vi "Dice Application.vi"() -> ()   [LabVIEW 2024]
uses:
  <vilib>/numeric/Random Number (Range) U64.vi
  <vilib>/numeric/sub_Random U32.vi
panel:
  out "Waveform Chart":u32(graph)
  in  "Throw Dice":bool
  in  "Stop":bool
  out "Dice":u32
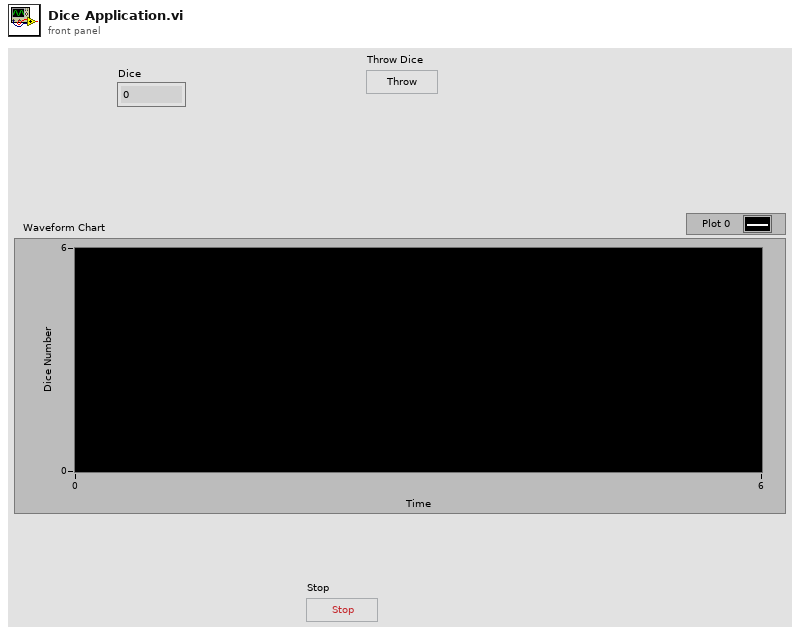
[diagram p1: front panel]
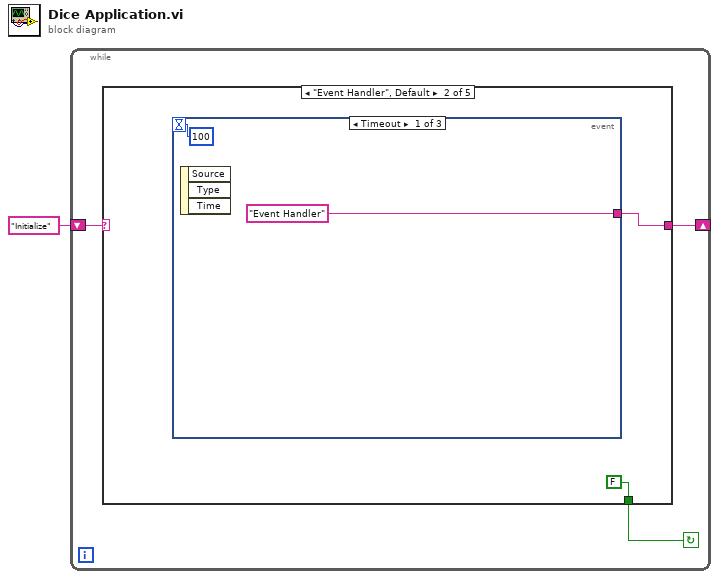
[diagram p0: block diagram]
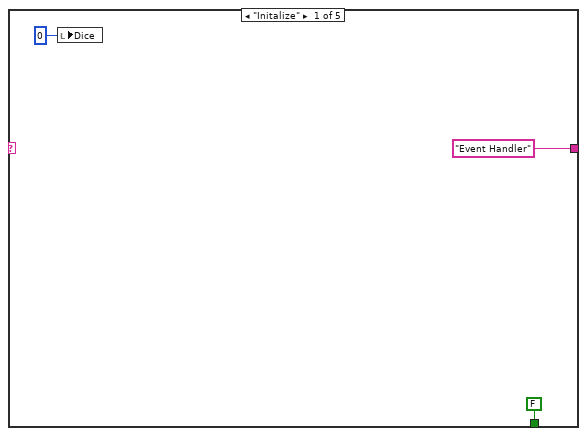
[diagram p2: hidden frame]
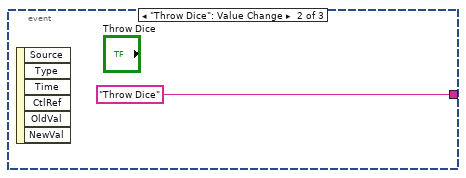
[diagram p3: hidden frame]
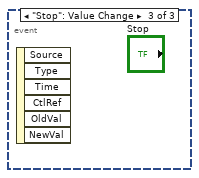
[diagram p4: hidden frame]
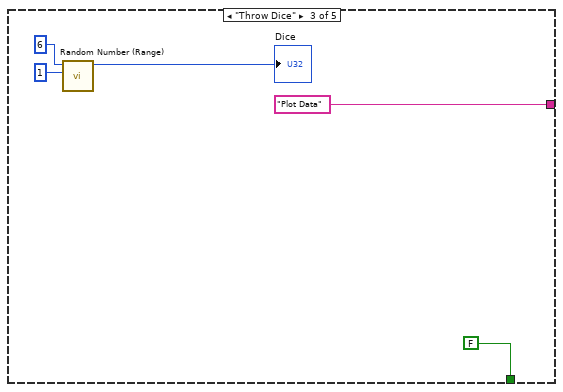
[diagram p5: hidden frame]
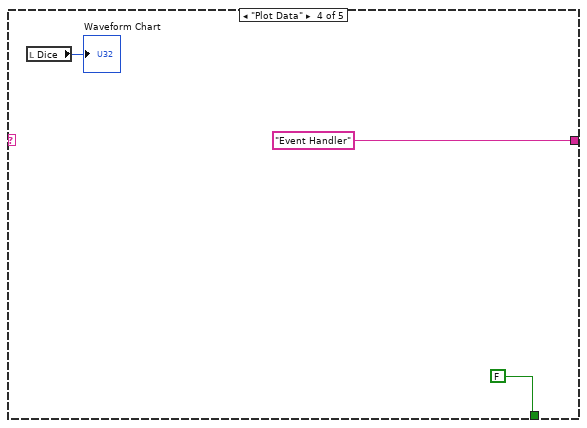
[diagram p6: hidden frame]
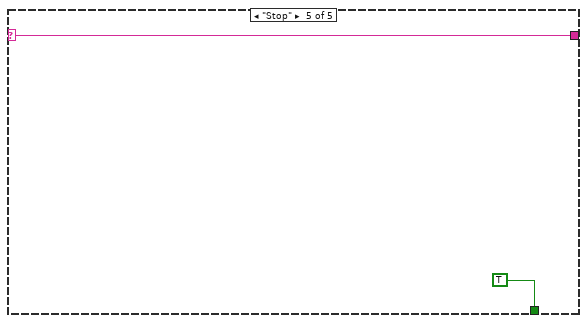
[diagram p7: hidden frame]
diagram:
  n1 = while {
    shift-right: [w3] -> _
    shift-left: "Initialize" -> [w4]
    stop <- w2 continue-if-true
    n2 = case shown="\"Event Handler\", Default" w4 {
      selector: w4 -> [_ _ _ _ w22]
      tunnel: ["Event Handler" w9 "Plot Data" "Event Handler" w22] -> w3
      tunnel: [FALSE FALSE FALSE FALSE TRUE] -> w2
      frame "Initalize" {
        n3 = local write "Dice"(u64 0 ("Dice")) -> ()
      }
      frame "Event Handler", Default {
        n4 = event shown="[0] Timeout" {
          selector: _ -> [_ _ _]
          dyn-events: _ -> [_ _ _]
          timeout: 100 -> [_ _ _]
          tunnel: ["Event Handler" "Throw Dice" _] -> w9
          event Timeout {
            n5 = event-data() -> ()  [unwired: 1 in, 3 out]
          }
          event "Throw Dice": Value Change {
            n6 = event-data() -> ()  [unwired: 1 in, 6 out]
          }
          event "Stop": Value Change {
            n7 = event-data() -> ()  [unwired: 1 in, 6 out]
          }
        }
      }
      frame "Throw Dice" {
        n8 = call-poly <vilib>:"Random Number (Range).vi"("lower bound (0)"=u64 1, "upper bound (100)"=u64 6) -> ("number"=→"Dice":u64)  [unwired: 9 in]
      }
      frame "Plot Data" {
        n9 = local read "Dice"() -> (→"Waveform Chart":u32)
      }
      frame "Stop" {
      }
    }
  }
